vi "SetOnlyDelaysHW.vi"(8 "error in (no error)":errorcluster, 11 "BME_DG_Base in":refnum<class "BME_DG_Base.lvclass">) -> (0 "error out":errorcluster, 3 "BME_DG_Base out":refnum<class "BME_DG_Base.lvclass">)   [LabVIEW 2009, in "POLARIS BME DG.lvlib" / "BME_DG_Base.lvclass"]
doc: "VIs calls ModifyChnlHW.vi of a channel class for each channel containing in objChnls. ModifyChnlHW.vi calls appropriate DLL function, Set_G02_Delay, Set_GO5_Delay, Set_G05P2_Delay or Set_G08_Delay.\n\n\nauthor: Alexander Kessler, Helmholtz-Institut-Jena \nmaintainer: Alexander Kessler: alexander.kessler@uni-jena.de\n\nLast Change:\nLicense Agreement for this software:\n\nCopyright (C)\nHelmholtz-Institut-Jena\nFröbelsteg 3\n07743 Jena\nGermany\n\nContact: alexander.kessler@uni-jena.de\n\nThis program is free software; you can redistribute it and/or modify it under the terms of the GNU General Public License as published by the Free Software Foundation; either version 2 of the license, or (at your option) any later version.\n\nThis program is distributed in the hope that it will be useful, but WITHOUT ANY WARRANTY; without even the implied warranty of MERCHANTABILITY or FITNESS FOR A PARTICULAR PURPOSE. See the GNU General License for more details (http://www.gnu.org)."
uses:
  BME_DG_Base.lvclass
  BME_DG_Base.lvclass/BME_DG_Base.ctl
  BME_DG_Chnl/BME_DG_Chnl.lvclass
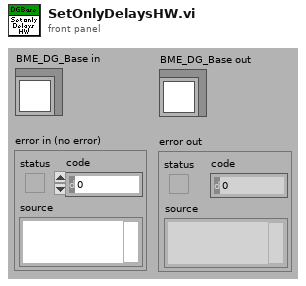
[diagram p1: front panel]
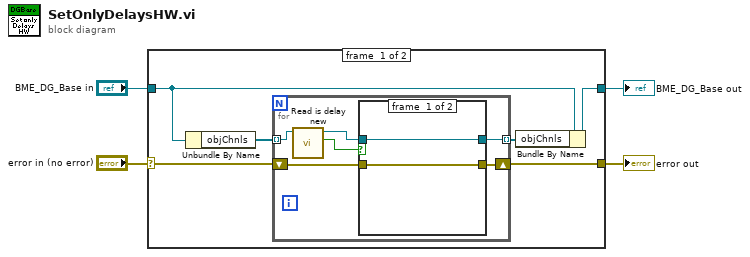
[diagram p0: block diagram]
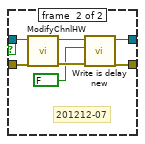
[diagram p2: hidden frame]
diagram:
  n1 = case shown="No Error" "error in (no error)" {
    selector: "error in (no error)" -> [w6 w27]
    tunnel: [w5 w27] -> w3
    tunnel: [w8 w26] -> w1
    tunnel: "BME_DG_Base in" -> [w10 w26]
    frame #0 {
      n2 = Unbundle By Name(w10) -> ("objChnls"=w9:refnum<class "BME_DG_Chnl.lvclass">[])
      n3 = for {
        tunnel: w9 -> [w13] mode=indexing
        tunnel: [w16] -> w7 mode=indexing
        shift-right: [w15] -> w5
        shift-left: w6 -> [w14]
        n4 = call "Read is delay new.vi"("BME_DG_Chnl in"=w13) -> ("Needs HW Update"=w11:bool, "BME_DG_Chnl out"=w12:refnum<class "BME_DG_Chnl.lvclass">)  [unwired: 8 in, 1 out]
        n5 = case shown="True" w11 {
          tunnel: w12 -> [w18 w25]
          tunnel: [w18 w20] -> w16
          tunnel: w14 -> [w17 w24]
          tunnel: [w17 w19] -> w15
          frame #0 {
          }
          frame #1 {
            # "201212-07"
            n6 = call-dynamic "ModifyChnlHW.vi"("error in (no error)"=w24, "BME_DG_Chnl in"=w25) -> ("error out"=w23:errorcluster, "BME_DG_Chnl out"=w22:refnum<class "BME_DG_Chnl.lvclass">)  [unwired: 8 in]
            n7 = call "Write is delay new.vi"("error in (no error)"=w23, "Needs HW Update"=FALSE, "BME_DG_Chnl in"=w22) -> ("error out"=w19:errorcluster, "BME_DG_Chnl out"=w20:refnum<class "BME_DG_Chnl.lvclass">)  [unwired: 7 in]
          }
        }
      }
      n8 = Bundle By Name(cluster=w10, "objChnls"=w7) -> (w8:refnum<class "BME_DG_Base.lvclass">)
    }
    frame #1 {
    }
  }
  "error out" <- w3
  "BME_DG_Base out" <- w1
